vi "CAENHVWrapper Example for SY4527-SY5527.vi"() -> ()   [LabVIEW 2009]
uses:
  <userlib>/CAENHVWrapper/Types/PARAM_MODE.ctl
  <userlib>/CAENHVWrapper/CAENHVWrapper.lvlib
panel:
  out "error":bool
  out "ok":bool
  out "error out":errorcluster
  in  "System Settings Button":bool
  in  "system_set_button":bool
  in  "sysparam_io":string
  in  "Parameters list":string(combo)
  in  "Select a command:":string(combo)
  in  "channel_set_button":bool
  in  "board_set_button":bool
  in  "System Load Button":bool
  in  "CHANNEL":u16
  in  "SLOT":u16
  in  "Params Refresh Button":bool
  in  "reset_ui":dbl
  in  "chparam_io":string
  in  "bdparam_io":string
  in  "Channel Parameters list":string(combo)
  in  "Board Parameters list":string(combo)
  out "NrOfSlot":u16
  in  "Crate Refresh Button":bool
  out "crate_map":string[][](table)
  in  "System Stop Button":bool
  in  "System Start Button":bool
  in  "Password":string="admin"
  in  "Username":string="admin"
  in  "IP Address":string="192.168.0.1"
  # "HVWrapper library\nFunctions Demo\nSY4527(LC) / SY5527(LC)"
  # "step\n1"
  # "step\n2"
  # "Connection"
  # "System parameters"
  # "Crate Map"
  # "Board and Channel parameters"
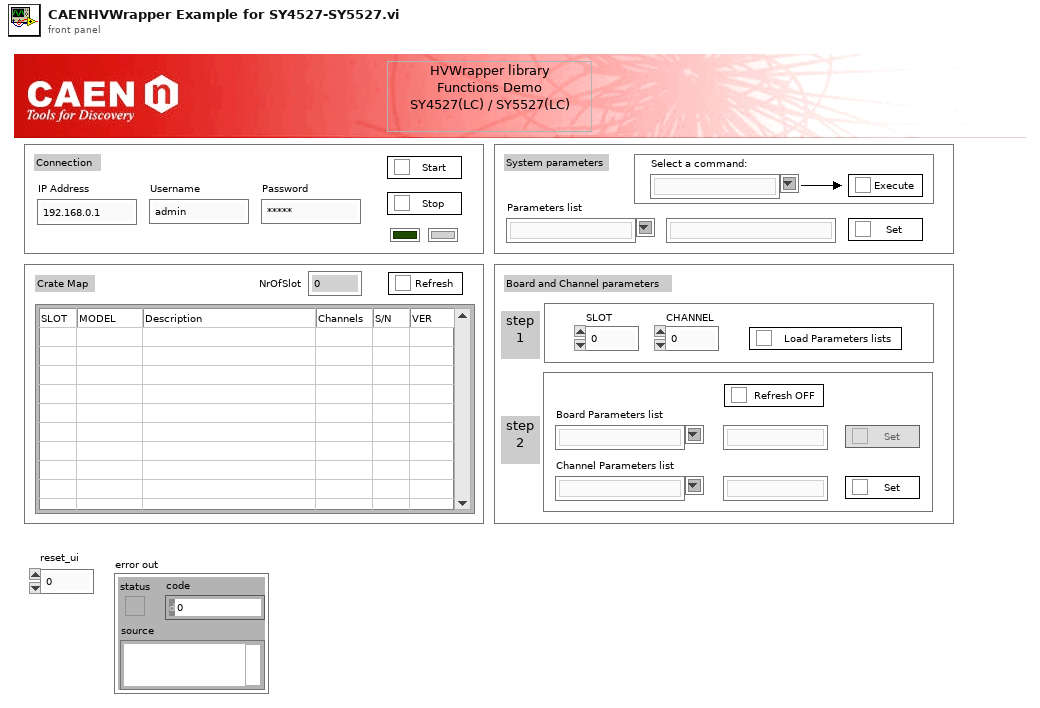
[diagram p1: front panel]
types:
  T1 = enum8{"Enabled", "Disabled", "Disabled and Grayed Out"}
  T2 = typedef "CAENHVWrapper.lvlib/PARAM_MODE.ctl" = enum32{"PARAM_MODE_RDONLY", "PARAM_MODE_WRONLY", "PARAM_MODE_RDWR"}
  T3 = typedef "CAENHVWrapper.lvlib/PARAM_TYPE.ctl" = enum32{"PARAM_TYPE_NUMERIC", "PARAM_TYPE_ONOFF", "PARAM_TYPE_CHSTATUS", "PARAM_TYPE_BDSTATUS", "PARAM_TYPE_BINARY", "PARAM_TYPE_STRING"}
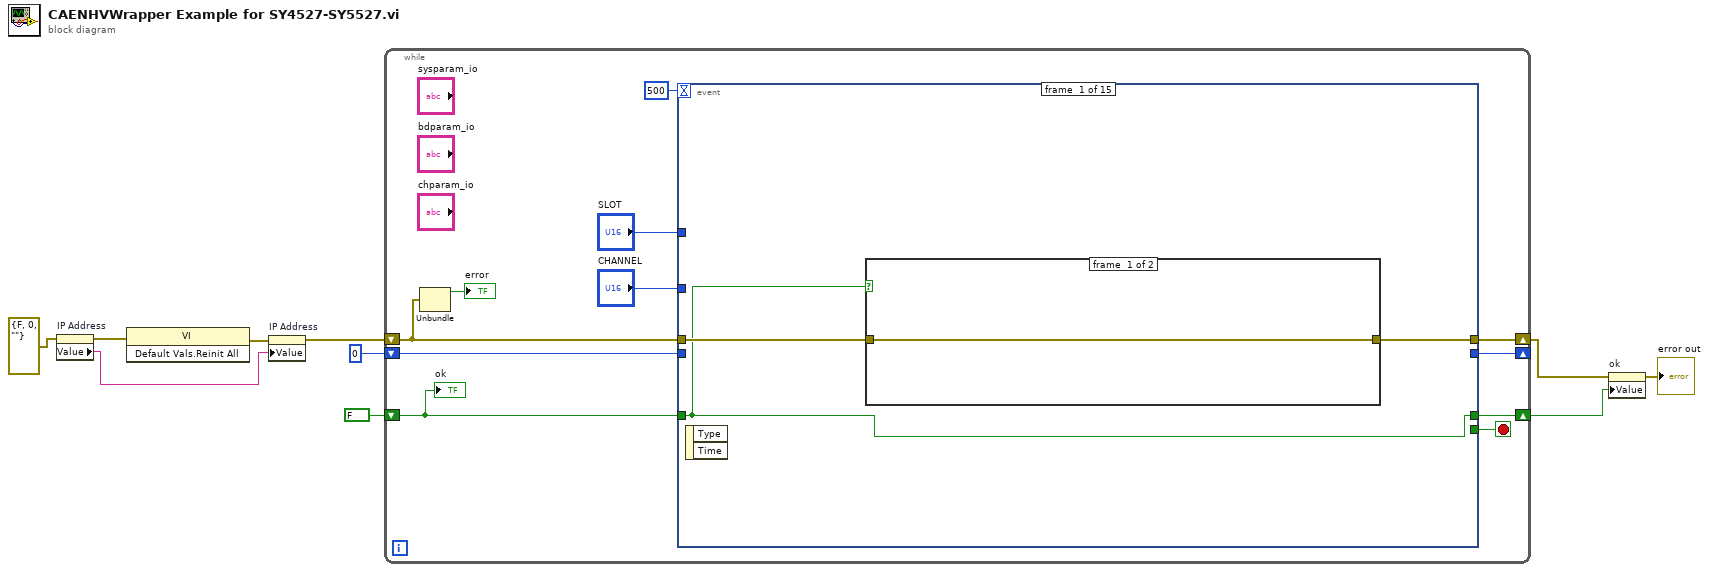
[diagram p0: block diagram]
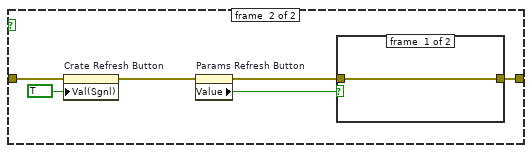
[diagram p2: hidden frame]
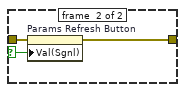
[diagram p3: hidden frame]
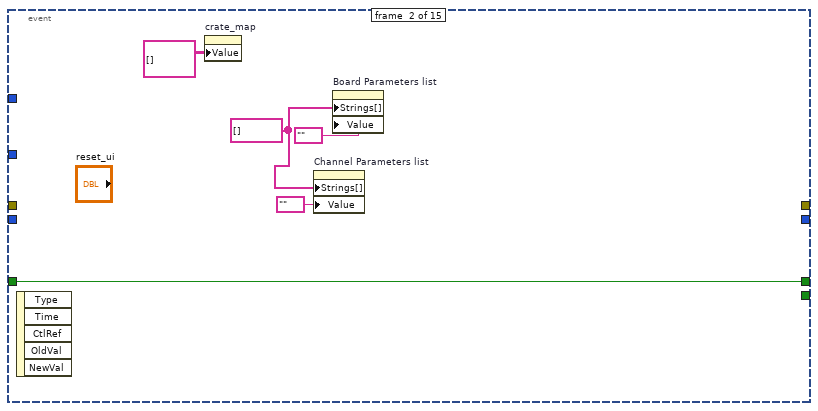
[diagram p4: hidden frame]
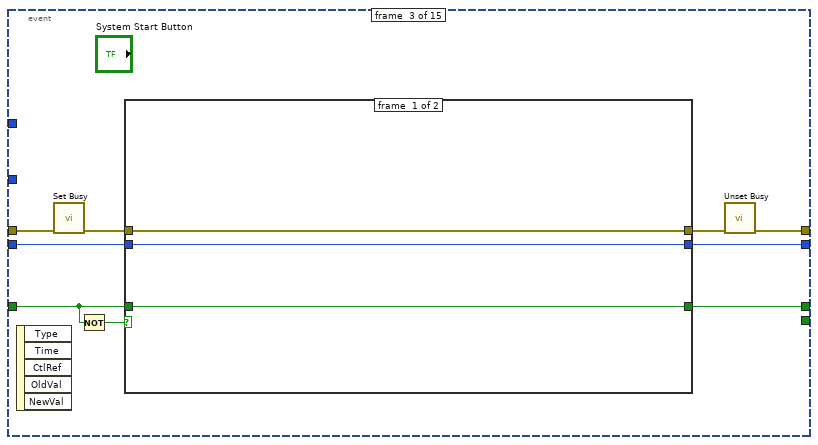
[diagram p5: hidden frame]
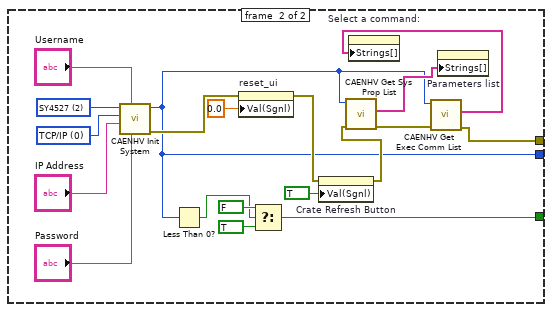
[diagram p6: hidden frame]
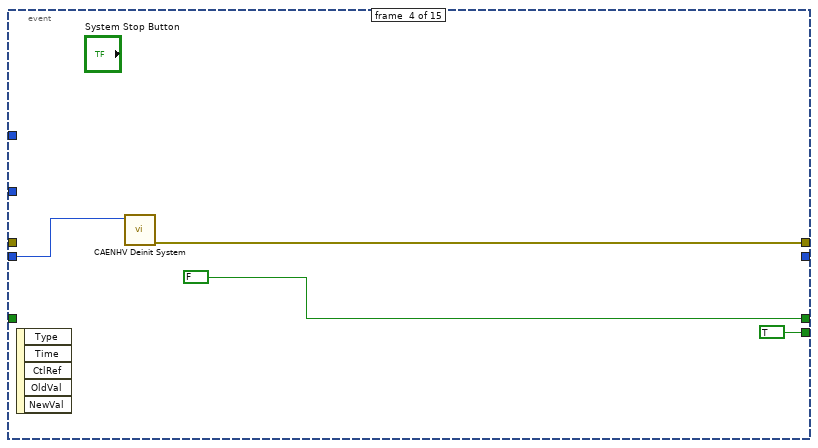
[diagram p7: hidden frame]
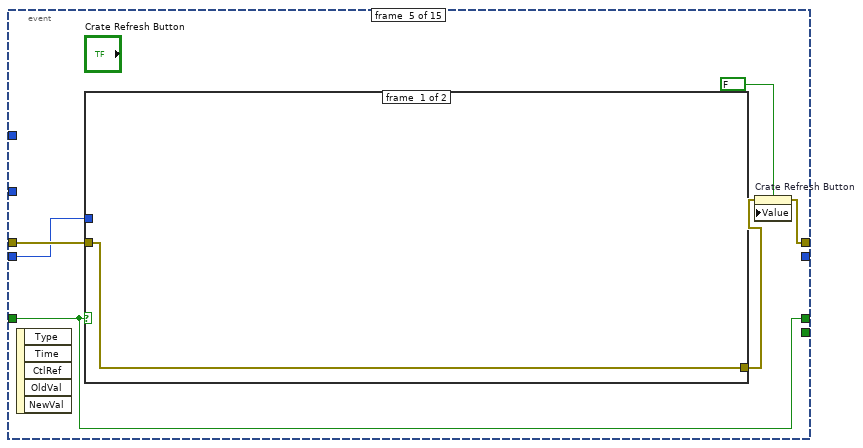
[diagram p8: hidden frame]
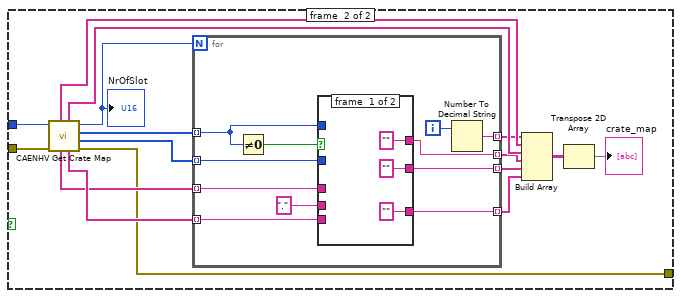
[diagram p9: hidden frame]
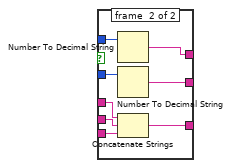
[diagram p10: hidden frame]
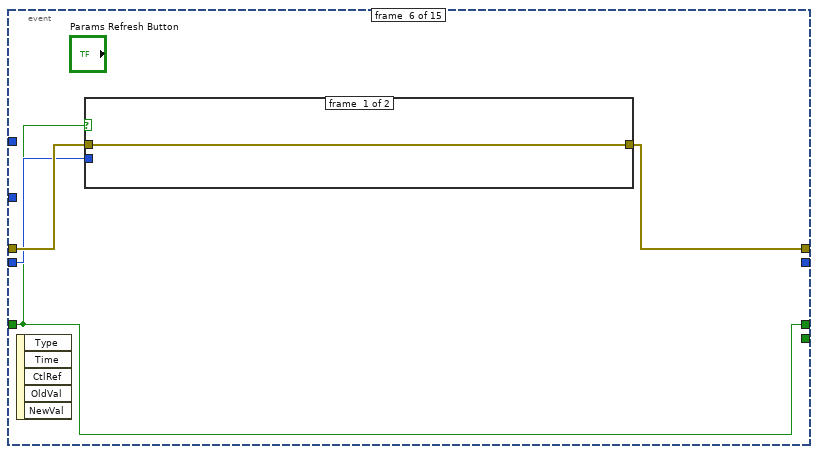
[diagram p11: hidden frame]
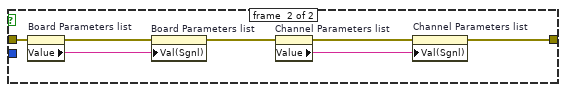
[diagram p12: hidden frame]
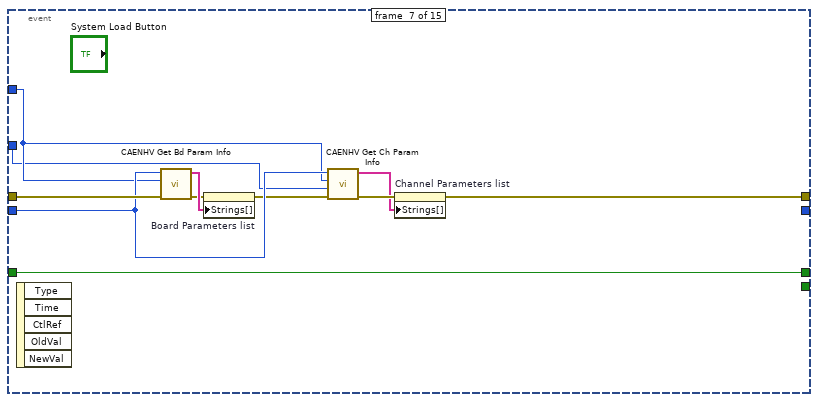
[diagram p13: hidden frame]
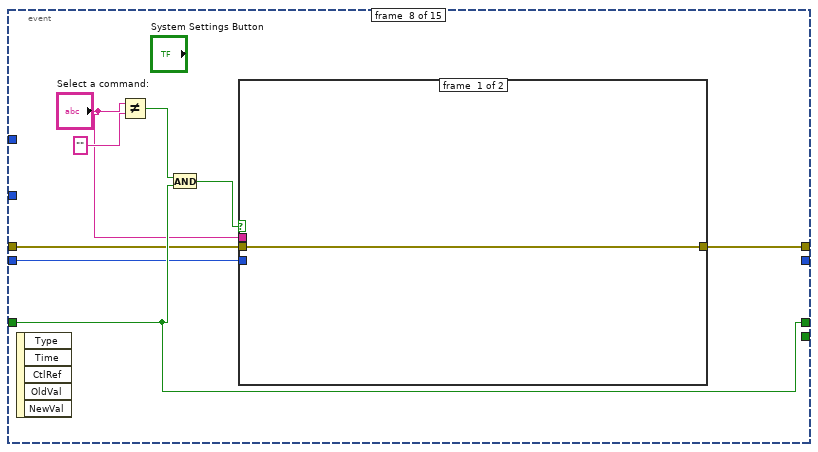
[diagram p14: hidden frame]
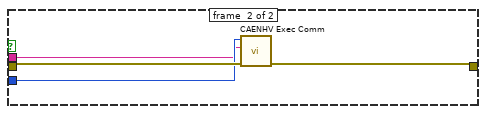
[diagram p15: hidden frame]
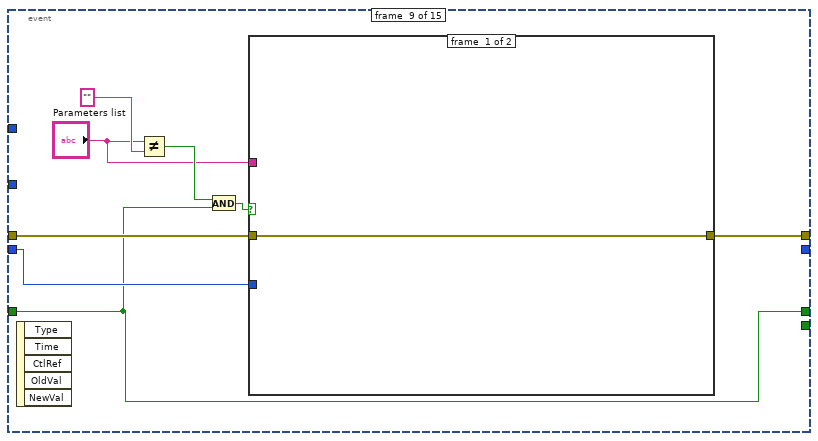
[diagram p16: hidden frame]
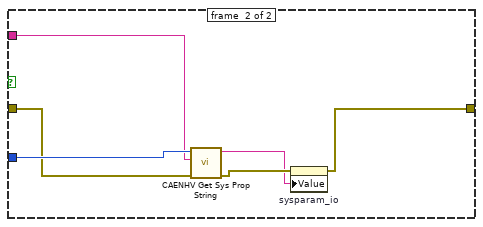
[diagram p17: hidden frame]
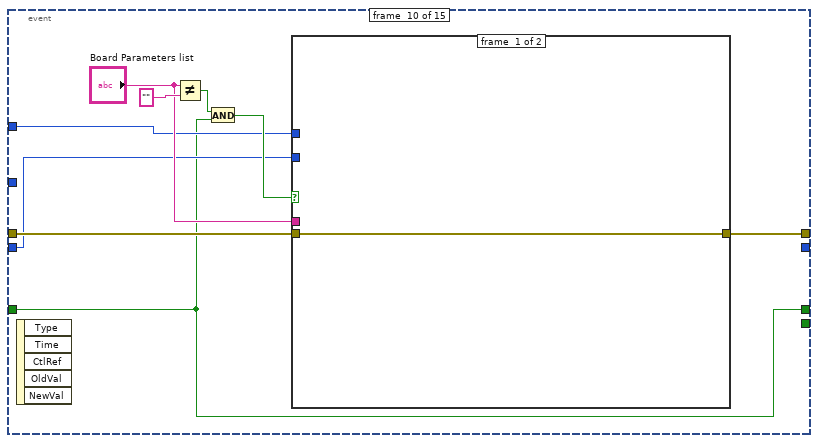
[diagram p18: hidden frame]
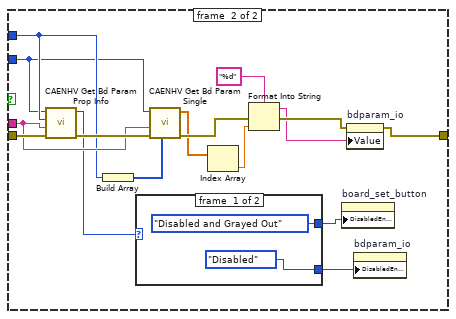
[diagram p19: hidden frame]
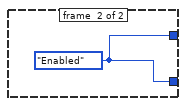
[diagram p20: hidden frame]
diagram:
  n1 = property on="IP Address" class="Str"(error in=errorcluster {"status"=FALSE, "code"=0, "source"=""} ("error out")) -> (error out=w5:errorcluster, "Value"=w2:string)  [unwired: 1 in, 1 out]
  n2 = invoke class="VI" method="Default Vals.Reinit All"(error in=w5) -> (error out=w4:errorcluster)  [unwired: 2 in, 2 out]
  n3 = property on="IP Address" class="Str"(error in=w4, "Value"=w2) -> (error out=w3:errorcluster)  [unwired: 1 in, 1 out]
  n4 = while {
    shift-right: [w20] -> _
    shift-left: 0 ("handle") -> [w18]
    shift-right: [w21] -> w1
    shift-left: w3 -> [w12]
    shift-right: [w19] -> w8
    shift-left: FALSE -> [w13]
    stop <- w17 stop-if-true
    n5 = Unbundle(w12) -> ("status"=→"error":bool)  [unwired: 2 out]
    n6 = event shown="[13] \"channel_set_button\": Value Change" {
      selector: _ -> [_ _ _ _ _ _ _ _ _ _ _ _ _ _ _]
      dyn-events: _ -> [_ _ _ _ _ _ _ _ _ _ _ _ _ _ _]
      timeout: 500 -> [_ _ _ _ _ _ _ _ _ _ _ _ _ _ _]
      tunnel: [w23 _ w41 w74 w78 w121 w133 w146 w162 w176 w206 w263 _ w280 _] -> w21
      tunnel: [_ _ w49 _ _ _ _ _ _ _ _ _ _ _ _] -> w20
      tunnel: [w22 w40 w48 FALSE w79 w122 w143 w148 w159 w172 w203 w265 _ w283 w328] -> w19
      tunnel: w13 -> [w22 w40 w46 _ w79 w122 w143 w148 w159 w172 w203 w265 _ w283 w328]
      tunnel: w12 -> [w24 _ w44 _ w81 w124 w142 w147 w164 w177 w207 w264 _ w281 _]
      tunnel: w18 -> [_ _ w45 w75 w80 w123 w141 w145 w163 w174 w205 w262 _ w279 _]
      tunnel: [_ _ _ TRUE _ _ _ _ _ _ _ _ _ _ _] -> w17
      tunnel: "SLOT" -> [_ _ _ _ _ _ w140 _ _ w173 w204 _ _ w278 _]
      tunnel: "CHANNEL" -> [_ _ _ _ _ _ w139 _ _ _ w202 _ _ w277 _]
      event #0 {
        n7 = event-data() -> ()  [unwired: 1 in, 2 out]
        n8 = case shown="True" w22 {
          tunnel: w24 -> [w25 w31]
          tunnel: [w25 w30] -> w23
          frame #0 {
          }
          frame #1 {
            n9 = property on="Crate Refresh Button" class="Bool (strict)"(error in=w31, "Val(Sgnl)"=TRUE ("Value (Signaling)")) -> (error out=w28:errorcluster)  [unwired: 1 in, 1 out]
            n10 = property on="Params Refresh Button" class="Bool (strict)"(error in=w28) -> (error out=w27:errorcluster, "Value"=w26:bool)  [unwired: 1 in, 1 out]
            n11 = case shown="True" w26 {
              selector: w26 -> [_ w33]
              tunnel: [w32 w35] -> w30
              tunnel: w27 -> [w32 w34]
              frame #0 {
              }
              frame #1 {
                n12 = property on="Params Refresh Button" class="Bool (strict)"(error in=w34, "Val(Sgnl)"=w33) -> (error out=w35:errorcluster)  [unwired: 1 in, 1 out]
              }
            }
          }
        }
      }
      event #1 {
        w38 = string[] [] ("Strings []")
        n13 = event-data() -> ()  [unwired: 1 in, 5 out]
        n14 = property on="crate_map" class="Tbl (strict)"("Value"=string[][] [] ("crate_map")) -> ()  [unwired: 2 in, 2 out]
        n15 = property on="Channel Parameters list" class="CmbBox"("Strings[]"=w38, "Value"="" ("Channel Parameters")) -> ()  [unwired: 2 in, 2 out]
        n16 = property on="Board Parameters list" class="CmbBox"("Strings[]"=w38, "Value"="" ("Board Parameters")) -> ()  [unwired: 2 in, 2 out]
      }
      event #2 {
        n17 = event-data() -> ()  [unwired: 1 in, 5 out]
        n18 = call <vilib>:"Set Busy.vi"("error in (no error)"=w44) -> ("error out"=w43:errorcluster)  [unwired: 9 in, 1 out]
        n19 = Not(x=w46) -> (.not. x?=w47:bool)
        n20 = case shown="True" w47 {
          tunnel: [w50 w53] -> w49
          tunnel: [w51 w67] -> w48
          tunnel: [w52 w61] -> w42
          tunnel: w43 -> [w52 _]
          tunnel: w46 -> [w51 _]
          tunnel: w45 -> [w50 _]
          frame #0 {
          }
          frame #1 {
            w64 = u32 2 items=["SY1527", "SY2527", "SY4527", "SY5527", "N568", "V65XX", "N1470", "V8100"] ("system")
            w68 = 0 items=["TCP/IP"=0, "HS CAENET"=2, "USB 2.0"=3, "CONET Optical Link"=4, "USB VCP"=5] ("LinkType")
            n21 = call <userlib>:"CAENHV Init System.vi"("Passwd"="Password", "UserName"="Username", "Arg"="IP Address", "LinkType"=w68, "system"=w64) -> ("error out"=w63:errorcluster, "handle"=w53:i32)  [unwired: 5 in]
            n22 = Less Than 0?(x=w53) -> (x < 0?=w54:bool)
            n23 = property on="reset_ui" class="DigNum (strict)"(error in=w63, "Val(Sgnl)"=0.0 ("Value (Signaling)")) -> (error out=w57:errorcluster)  [unwired: 1 in, 1 out]
            n24 = Select(t=FALSE, s=w54, f=TRUE) -> (s? t:f=w67:bool)
            n25 = property on="Crate Refresh Button" class="Bool (strict)"(error in=w57, "Val(Sgnl)"=TRUE ("Value (Signaling)")) -> (error out=w56:errorcluster)  [unwired: 1 in, 1 out]
            n26 = call <userlib>:"CAENHV Get Sys Prop List.vi"("error in (no error)"=w56, "handle"=w53) -> ("error out"=w62:errorcluster, "PropNameList"=w59:string[])  [unwired: 7 in, 1 out]
            n27 = call <userlib>:"CAENHV Get Exec Comm List.vi"("error in (no error)"=w62, "handle"=w53) -> ("error out"=w61:errorcluster, "CommNameList"=w58:string[])  [unwired: 7 in, 1 out]
            n28 = property on="Select a command:" class="CmbBox"("Strings[]"=w58) -> ()  [unwired: 2 in, 2 out]
            n29 = property on="Parameters list" class="CmbBox"("Strings[]"=w59) -> ()  [unwired: 2 in, 2 out]
          }
        }
        n30 = call <vilib>:"Unset Busy.vi"("error in (no error)"=w42) -> ("error out"=w41:errorcluster)  [unwired: 10 in]
      }
      event #3 {
        n31 = event-data() -> ()  [unwired: 1 in, 5 out]
        n32 = call <userlib>:"CAENHV Deinit System.vi"("handle"=w75) -> ("error out"=w74:errorcluster)  [unwired: 10 in]
      }
      event #4 {
        n33 = event-data() -> ()  [unwired: 1 in, 5 out]
        n34 = case shown="True" w79 {
          tunnel: w81 -> [w82 w98]
          tunnel: w80 -> [_ w97]
          tunnel: [w82 w83] -> w77
          frame #0 {
          }
          frame #1 {
            n35 = call <userlib>:"CAENHV Get Crate Map.vi"("error in (no error)"=w98, "handle"=w97) -> ("error out"=w83:errorcluster, "SerNumList"=w88:i16[], "NrofChList"=w92:i16[], "NrOfSlot"=w94:u16, "FmwRelMinList"=w86:string[], "DescriptionList"=w95:string[], "FmwRelMaxList"=w85:string[], "ModelList"=w96:string[])  [unwired: 2 in]
            "NrOfSlot" <- w94
            n36 = for {
              N: w94 -> [_]
              tunnel: [w100] -> w93 mode=indexing
              tunnel: w92 -> [w102] mode=indexing
              tunnel: [w109] -> w91 mode=indexing
              tunnel: w88 -> [w108] mode=indexing
              tunnel: [w107] -> w87 mode=indexing
              tunnel: w86 -> [w104] mode=indexing
              tunnel: w85 -> [w106] mode=indexing
              tunnel: [w105] -> w84 mode=indexing
              i -> [w99]
              n37 = Not Equal To 0?(x=w102) -> (x != 0?=w101:bool)
              n38 = case shown="False" w101 {
                tunnel: ["" w120] -> w109
                tunnel: w108 -> [_ w119]
                tunnel: ["" w118] -> w107
                tunnel: w106 -> [_ w117]
                tunnel: ["" w116] -> w105
                tunnel: w104 -> [_ w115]
                tunnel: "." ("string") -> [_ w114]
                tunnel: w102 -> [_ w113]
                frame #0 {
                }
                frame #1 {
                  n39 = Number To Decimal String(number=w113) -> (decimal integer string=w120:string)  [unwired: 1 in]
                  n40 = Number To Decimal String(number=w119) -> (decimal integer string=w118:string)  [unwired: 1 in]
                  n41 = Concatenate Strings(w117, w114, w115) -> (w116:string)
                }
              }
              n42 = Number To Decimal String(number=w99) -> (decimal integer string=w100:string)  [unwired: 1 in]
            }
            n43 = Build Array(w93, w96, w95, w91, w87, w84) -> (w90:string[][])
            n44 = Transpose 2D Array(2D array=w90) -> (transposed array=→"crate_map":string[][])
          }
        }
        n45 = property on="Crate Refresh Button" class="Bool (strict)"(error in=w77, "Value"=FALSE ("System Refresh Button")) -> (error out=w78:errorcluster)  [unwired: 1 in, 1 out]
      }
      event #5 {
        n46 = event-data() -> ()  [unwired: 1 in, 5 out]
        n47 = case shown="True" w122 {
          tunnel: w124 -> [w125 w130]
          tunnel: w123 -> [_ _]
          tunnel: [w125 w126] -> w121
          frame #0 {
          }
          frame #1 {
            n48 = property on="Board Parameters list" class="CmbBox"(error in=w130) -> (error out=w131:errorcluster, "Value"=w132:string)  [unwired: 1 in, 1 out]
            n49 = property on="Board Parameters list" class="CmbBox"(error in=w131, "Val(Sgnl)"=w132) -> (error out=w129:errorcluster)  [unwired: 1 in, 1 out]
            n50 = property on="Channel Parameters list" class="CmbBox"(error in=w129) -> (error out=w127:errorcluster, "Value"=w128:string)  [unwired: 1 in, 1 out]
            n51 = property on="Channel Parameters list" class="CmbBox"(error in=w127, "Val(Sgnl)"=w128) -> (error out=w126:errorcluster)  [unwired: 1 in, 1 out]
          }
        }
      }
      event #6 {
        n52 = event-data() -> ()  [unwired: 1 in, 5 out]
        n53 = call <userlib>:"CAENHV Get Bd Param Info.vi"("error in (no error)"=w142, "slot"=w140, "handle"=w141) -> ("error out"=w137:errorcluster, "ParNameList"=w138:string[])  [unwired: 7 in]
        n54 = property on="Board Parameters list" class="CmbBox"(error in=w137, "Strings[]"=w138) -> (error out=w136:errorcluster)  [unwired: 1 in, 1 out]
        n55 = call <userlib>:"CAENHV Get Ch Param Info.vi"("error in (no error)"=w136, "Ch"=w139, "slot"=w140, "handle"=w141) -> ("error out"=w135:errorcluster, "ParNameList"=w134:string[])  [unwired: 5 in, 1 out]
        n56 = property on="Channel Parameters list" class="CmbBox"(error in=w135, "Strings[]"=w134) -> (error out=w133:errorcluster)  [unwired: 1 in, 1 out]
      }
      event #7 {
        n57 = event-data() -> ()  [unwired: 1 in, 5 out]
        n58 = Not Equal?(x="Select a command:", y="") -> (x != y?=w150:bool)
        n59 = And(x=w150, y=w148) -> (x .and. y?=w149:bool)
        n60 = case shown="True" w149 {
          tunnel: w147 -> [w152 w156]
          tunnel: [w152 w155] -> w146
          tunnel: w145 -> [_ w154]
          tunnel: "Select a command:" -> [_ w153]
          frame #0 {
          }
          frame #1 {
            n61 = call <userlib>:"CAENHV Exec Comm.vi"("error in (no error)"=w156, "CommName"=w153, "handle"=w154) -> ("error out"=w155:errorcluster)  [unwired: 8 in]
          }
        }
      }
      event #8 {
        n62 = event-data() -> ()  [unwired: 1 in, 5 out]
        n63 = Not Equal?(x="Parameters list", y="") -> (x != y?=w160:bool)
        n64 = And(x=w160, y=w159) -> (x .and. y?=w158:bool)
        n65 = case shown="True" w158 {
          tunnel: w164 -> [w165 w170]
          tunnel: w163 -> [_ w171]
          tunnel: [w165 w168] -> w162
          tunnel: "Parameters list" -> [_ w166]
          frame #0 {
          }
          frame #1 {
            n66 = call <userlib>:"CAENHV Get Sys Prop String.vi"("error in (no error)"=w170, "PropName"=w166, "handle"=w171) -> ("error out"=w169:errorcluster, "Result"=w167:string)  [unwired: 7 in]
            n67 = property on="sysparam_io" class="Str"(error in=w169, "Value"=w167) -> (error out=w168:errorcluster)  [unwired: 1 in, 1 out]
          }
        }
      }
      event #9 {
        n68 = event-data() -> ()  [unwired: 1 in, 5 out]
        n69 = Not Equal?(x="Board Parameters list", y="") -> (x != y?=w179:bool)
        n70 = And(x=w179, y=w172) -> (x .and. y?=w178:bool)
        n71 = case shown="True" w178 {
          tunnel: w177 -> [w181 w189]
          tunnel: [w181 w193] -> w176
          tunnel: "Board Parameters list" -> [_ w187]
          tunnel: w174 -> [_ w185]
          tunnel: w173 -> [_ w186]
          frame #0 {
          }
          frame #1 {
            n72 = call <userlib>:"CAENHV Get Bd Param Prop Info.vi"("error in (no error)"=w189, "ParName"=w187, "slot"=w186, "handle"=w185) -> ("error out"=w188:errorcluster, "PropMode"=w184:T2)  [unwired: 5 in, 1 out]
            n73 = Build Array(w186) -> (w192:u16[])
            n74 = case shown="\"PARAM_MODE_RDONLY\"" w184 {
              tunnel: [T1."Disabled and Grayed Out" ("Disabled") w200] -> w182
              tunnel: [T1."Disabled" ("Disabled") w200] -> w183
              frame #0 {
              }
              frame #1 {
                w200 = T1."Enabled" ("Disabled")
              }
            }
            n75 = call <userlib>:"CAENHV Get Bd Param Single.vi"("slotList"=w192, "error in (no error)"=w188, "ParName"=w187, "handle"=w185) -> ("error out"=w196:errorcluster, "ParValList"=w191:sgl[])  [unwired: 6 in]
            n76 = Index Array(array=w191) -> (element=w190:sgl)  [unwired: 1 in]
            n77 = Format Into String(format string="%d", error in=w196, w190) -> (resulting string=w194:string, error out=w195:errorcluster)  [unwired: 1 in]
            n78 = property on="board_set_button" class="Bool"("DisabledEnum"=w182) -> ()  [unwired: 2 in, 2 out]
            n79 = property on="bdparam_io" class="Str"(error in=w195, "Value"=w194) -> (error out=w193:errorcluster)  [unwired: 1 in, 1 out]
            n80 = property on="bdparam_io" class="Str"("DisabledEnum"=w183) -> ()  [unwired: 2 in, 2 out]
          }
        }
      }
      event #10 {
        n81 = event-data() -> ()  [unwired: 1 in, 5 out]
        n82 = Not Equal?(x="Channel Parameters list", y="") -> (x != y?=w209:bool)
        n83 = And(x=w209, y=w203) -> (x .and. y?=w208:bool)
        n84 = case shown="True" w208 {
          tunnel: w207 -> [w211 w223]
          tunnel: [w211 w224] -> w206
          tunnel: "Channel Parameters list" -> [_ w222]
          tunnel: w205 -> [_ w220]
          tunnel: w204 -> [_ w215]
          tunnel: w202 -> [_ w218]
          tunnel: "Channel Parameters list" -> [_ w219]
          frame #0 {
          }
          frame #1 {
            n85 = call <userlib>:"CAENHV Get Ch Param Prop Info.vi"("ParName"=w222, "error in (no error)"=w223, "Ch"=w218, "slot"=w215, "handle"=w220) -> ("error out"=w221:errorcluster, "PARAM_TYPE"=w217:T3, "PARAM_MODE"=w214:T2)  [unwired: 4 in]
            n86 = Build Array(w218) -> (w216:u16[])
            n87 = case shown="\"PARAM_TYPE_NUMERIC\", Default" w217 {
              tunnel: [w239 w241 w251] -> w226
              tunnel: [w238 w242 w252] -> w225
              tunnel: w221 -> [w236 w250 w260]
              tunnel: w220 -> [w232 w247 w257]
              tunnel: w219 -> [w234 w249 w259]
              tunnel: w216 -> [w231 w246 w256]
              tunnel: w215 -> [w230 w248 w258]
              frame #0 {
                n88 = call <userlib>:"CAENHV Get Ch Param Single.vi"("ChList"=w231, "error in (no error)"=w236, "ParName"=w234, "slot"=w230, "handle"=w232) -> ("error out"=w235:errorcluster, "ParValList"=w233:sgl[])  [unwired: 5 in]
                n89 = Index Array(array=w233) -> (element=w237:sgl)  [unwired: 1 in]
                n90 = Format Into String(format string="%.1f", error in=w235, w237) -> (resulting string=w238:string, error out=w239:errorcluster)  [unwired: 1 in]
              }
              frame #1 {
                n91 = call <userlib>:"CAENHV Get Ch Param Bool.vi"("ChList"=w246, "error in (no error)"=w250, "ParName"=w249, "slot"=w248, "handle"=w247) -> ("error out"=w241:errorcluster, "ParValList"=w245:bool[])  [unwired: 5 in]
                n92 = Index Array(array=w245) -> (element=w244:bool)  [unwired: 1 in]
                n93 = Boolean To (0,1)(Boolean=w244) -> (0, 1=w243:i16)
                n94 = Number To Decimal String(number=w243) -> (decimal integer string=w242:string)  [unwired: 1 in]
              }
              frame #2 {
                n95 = call <userlib>:"CAENHV Get Ch Param Bool.vi"("ChList"=w256, "error in (no error)"=w260, "ParName"=w259, "slot"=w258, "handle"=w257) -> ("error out"=w251:errorcluster, "ParValList"=w255:bool[])  [unwired: 5 in]
                n96 = Index Array(array=w255) -> (element=w254:bool)  [unwired: 1 in]
                n97 = Boolean To (0,1)(Boolean=w254) -> (0, 1=w253:i16)
                n98 = Number To Decimal String(number=w253) -> (decimal integer string=w252:string)  [unwired: 1 in]
              }
            }
            n99 = case shown="\"PARAM_MODE_RDONLY\"" w214 {
              tunnel: [T1."Disabled and Grayed Out" ("Disabled") w229] -> w213
              tunnel: [T1."Disabled" ("Disabled") w229] -> w212
              frame #0 {
              }
              frame #1 {
                w229 = T1."Enabled" ("Disabled")
              }
            }
            n100 = property on="chparam_io" class="Str"("DisabledEnum"=w212) -> ()  [unwired: 2 in, 2 out]
            n101 = property on="channel_set_button" class="Bool"("DisabledEnum"=w213) -> ()  [unwired: 2 in, 2 out]
            n102 = property on="chparam_io" class="Str"(error in=w226, "Value"=w225) -> (error out=w224:errorcluster)  [unwired: 1 in, 1 out]
          }
        }
      }
      event #11 {
        n103 = event-data() -> ()  [unwired: 1 in, 5 out]
        n104 = property on="Parameters list" class="CmbBox"() -> ("Value"=w261:string)  [unwired: 2 in, 2 out]
        n105 = Not Equal?(x=w261, y="") -> (x != y?=w267:bool)
        n106 = And(x=w267, y=w265) -> (x .and. y?=w266:bool)
        n107 = case shown="True" w266 {
          tunnel: w264 -> [w269 w273]
          tunnel: [w269 w274] -> w263
          tunnel: w262 -> [_ w272]
          tunnel: w261 -> [_ w271]
          frame #0 {
          }
          frame #1 {
            n108 = property on="sysparam_io" class="Str"() -> ("Value"=w270:string)  [unwired: 2 in, 2 out]
            n109 = call <userlib>:"CAENHV Set Sys Prop String.vi"("error in (no error)"=w273, "Set"=w270, "PropName"=w271, "handle"=w272) -> ("error out"=w274:errorcluster)  [unwired: 7 in]
          }
        }
      }
      event #12 {
        n110 = event-data() -> ()  [unwired: 1 in, 5 out]
      }
      event #13 {
        n111 = event-data() -> ()  [unwired: 1 in, 5 out]
        n112 = property on="Channel Parameters list" class="CmbBox"() -> ("Value"=w276:string)  [unwired: 2 in, 2 out]
        n113 = Not Equal?(x=w276, y="") -> (x != y?=w284:bool)
        n114 = And(x=w284, y=w283) -> (x .and. y?=w282:bool)
        n115 = case shown="True" w282 {
          tunnel: w281 -> [w285 w298]
          tunnel: [w285 w293] -> w280
          tunnel: w279 -> [_ w291]
          tunnel: w278 -> [_ w290]
          tunnel: w277 -> [_ w288]
          tunnel: w276 -> [_ w289]
          frame #0 {
          }
          frame #1 {
            n116 = call <userlib>:"CAENHV Get Ch Param Prop Info.vi"("ParName"=w289, "error in (no error)"=w298, "Ch"=w288, "slot"=w290, "handle"=w291) -> ("error out"=w294:errorcluster, "PARAM_TYPE"=w292:T3, "PARAM_MODE"=w297:T2)  [unwired: 4 in]
            n117 = property on="chparam_io" class="Str"() -> ("Value"=w286:string)  [unwired: 2 in, 2 out]
            n118 = Build Array(w288) -> (w287:u16[])
            n119 = Equal?(x=w297, y=PARAM_MODE."PARAM_MODE_RDWR") -> (x = y?=w295:bool)
            n120 = case shown="True" w295 {
              tunnel: w294 -> [w299 w306]
              tunnel: [w299 w305] -> w293
              tunnel: w292 -> [_ w307]
              tunnel: w291 -> [_ w304]
              tunnel: w290 -> [_ w303]
              tunnel: w289 -> [_ w302]
              tunnel: w287 -> [_ w301]
              tunnel: w286 -> [_ w300]
              frame #0 {
              }
              frame #1 {
                n121 = case shown="\"PARAM_TYPE_ONOFF\"" w307 {
                  tunnel: w306 -> [w316 w325]
                  tunnel: [w315 w324] -> w305
                  tunnel: w304 -> [w314 w318]
                  tunnel: w303 -> [w313 w321]
                  tunnel: w302 -> [w312 w319]
                  tunnel: w301 -> [w311 w320]
                  tunnel: w300 -> [w309 w327]
                  frame #0 {
                    n122 = Scan Value(string=w309, format string="%f") -> (value=w308:dbl)  [unwired: 1 in, 1 out]
                    n123 = call <userlib>:"CAENHV Set Ch Param Single.vi"("ParValue"=w308, "ChList"=w311, "error in (no error)"=w316, "ParName"=w312, "slot"=w313, "handle"=w314) -> ("error out"=w315:errorcluster)  [unwired: 5 in]
                  }
                  frame #1 {
                    n124 = Scan Value(string=w327, format string="%d") -> (value=w323:dbl)  [unwired: 1 in, 1 out]
                    n125 = Equal?(x=1.0, y=w323) -> (x = y?=w322:bool)
                    n126 = call <userlib>:"CAENHV Set Ch Param Bool.vi"("ParValue"=w322, "ChList"=w320, "error in (no error)"=w325, "ParName"=w319, "slot"=w321, "handle"=w318) -> ("error out"=w324:errorcluster)  [unwired: 5 in]
                  }
                }
              }
            }
          }
        }
      }
      event #14 {
        n127 = event-data() -> ()  [unwired: 1 in, 6 out]
        n128 = property on="Params Refresh Button" class="Bool (strict)"("Val(Sgnl)"=FALSE ("Value (Signaling)")) -> ()  [unwired: 2 in, 2 out]
      }
    }
    "ok" <- w13
  }
  n129 = property on="ok" class="Bool (strict)"(error in=w1, "Value"=w8) -> (error out=→"error out":errorcluster)  [unwired: 1 in, 1 out]
